vi "Allosense - File to AWS Athena Converter.vi"() -> ()   [LabVIEW 2020]
uses:
  subvis/TimestampAction.ctl
  <vilib>/Utility/file.llb/Read Delimited Spreadsheet (string).vi
  <vilib>/Utility/file.llb/Write Delimited Spreadsheet (string).vi
panel:
  out "Status":string
  in  "Quick Save":bool
  in  "Save Header Settings":bool=TRUE
  in  "Load Header Settings":bool
  in  "Next 2":bool
  in  "Timing":T2(array[cluster])
  in  "Next":bool
  in  "Header Elements":T3(array[cluster])
  in  "Remove Header":bool=TRUE
  in  "Delimiter":string=","
  out "File Contents":string[][](array[string])
  # "Outputs:\n1. Updated .CSV (Timestamp Formatted)\n2. Header Datatype Table .TXT (for AWS Athena)\n3. Saved Header Configurations .BIN"
  # "OPTIONS"
  # "->"
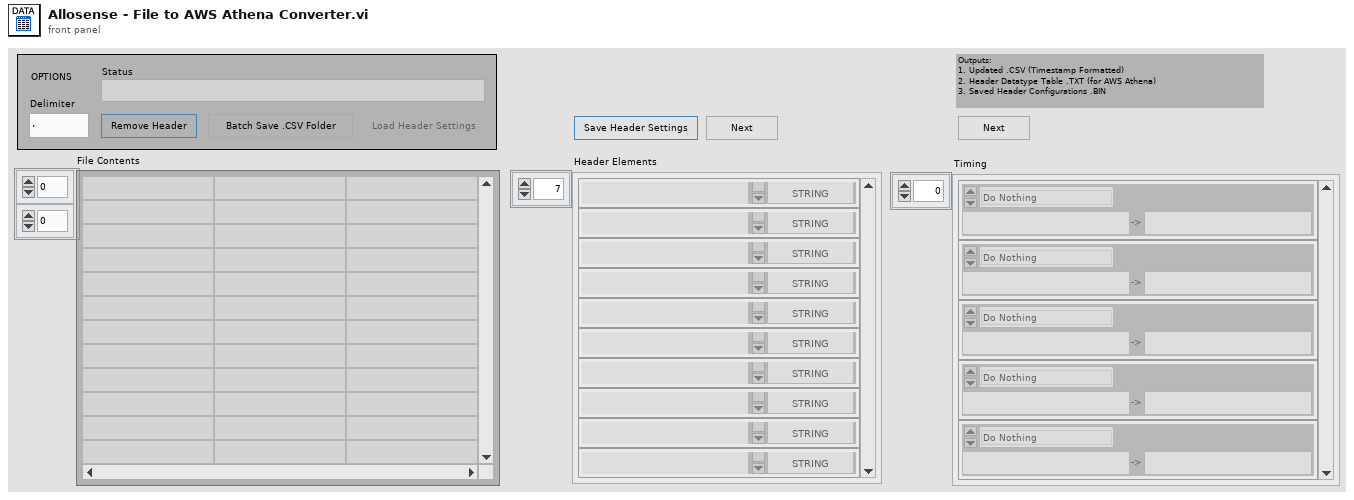
[diagram p1: front panel]
types:
  T1 = typedef "TimestampAction.ctl" = enum16{"Do Nothing", "Remove T"}
  T2 = cluster{"Original":string, "Action":T1, "Processed":string}[]
  T3 = cluster{"Item Name":string, "Item Type":enum16{"STRING", "TINYINT", "SMALLINT", "INT", "BIGINT", "BOOLEAN", "FLOAT", "DOUBLE", "DECIMAL", "ARRAY", "MAP", "TIMESTAMP", "DATE"}}[]
  T4 = enum16{"STRING", "TINYINT", "SMALLINT", "INT", "BIGINT", "BOOLEAN", "FLOAT", "DOUBLE", "DECIMAL", "ARRAY", "MAP", "TIMESTAMP", "DATE"}
  T5 = cluster{"Item Name":string, "Item Type":enum16{"STRING", "TINYINT", "SMALLINT", "INT", "BIGINT", "BOOLEAN", "FLOAT", "DOUBLE", "DECIMAL", "ARRAY", "MAP", "TIMESTAMP", "DATE"}}
  T6 = cluster{"Original":string, "Action":T1, "Processed":string}
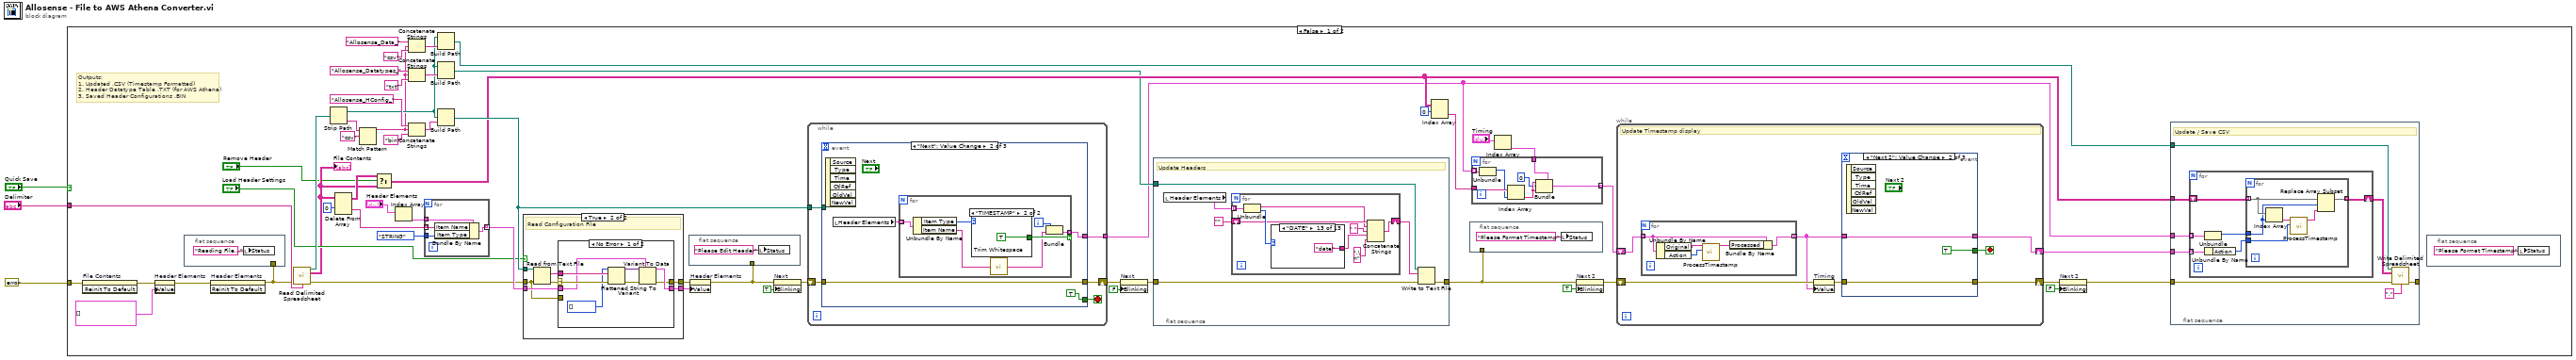
[diagram p0: block diagram]
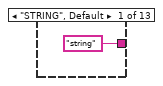
[diagram p2: hidden frame]
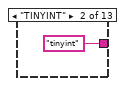
[diagram p3: hidden frame]
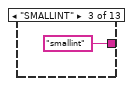
[diagram p4: hidden frame]
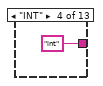
[diagram p5: hidden frame]
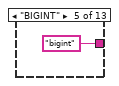
[diagram p6: hidden frame]
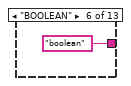
[diagram p7: hidden frame]
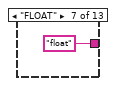
[diagram p8: hidden frame]
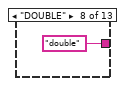
[diagram p9: hidden frame]
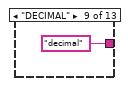
[diagram p10: hidden frame]
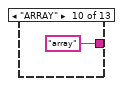
[diagram p11: hidden frame]
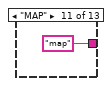
[diagram p12: hidden frame]
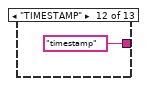
[diagram p13: hidden frame]
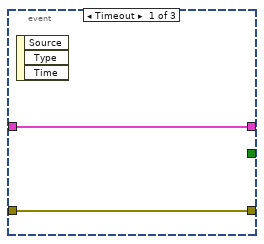
[diagram p14: hidden frame]
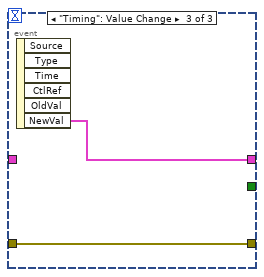
[diagram p15: hidden frame]
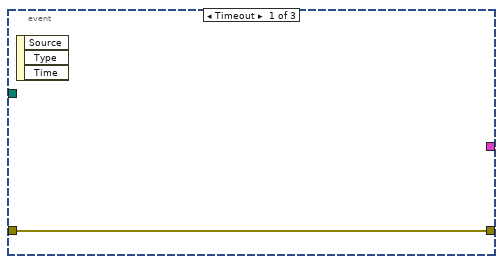
[diagram p16: hidden frame]
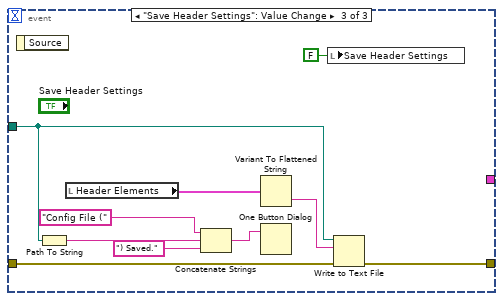
[diagram p18: hidden frame]
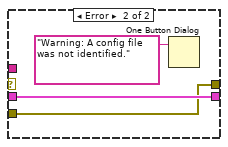
[diagram p20: hidden frame]
diagram:
  n1 = case shown="False" "Quick Save" {
    tunnel: errorcluster {"status"=FALSE, "code"=0, "source"=""} ("error in (no error)") -> [w8 w197]
    tunnel: "Delimiter" -> [w7 w189]
    frame False {
      # "Outputs:\n1. Updated .CSV (Timestamp Formatted)\n2. Header Datatype Table .TXT (for AWS Athena)\n3. Saved Header Configurations .BIN"
      n2 = invoke on="File Contents" class="Arr (strict)" method="Reinit To Default"(error in=w8) -> (error out=w57:errorcluster)  [unwired: 2 in, 2 out]
      n3 = property on="Header Elements" class="Arr (strict)"(error in=w57, "Value"=T3 [] ("Header Elements")) -> (error out=w56:errorcluster)  [unwired: 1 in, 1 out]
      n4 = flat-sequence {
        tunnel: w6 -> [_]
        frame #0 {
          n5 = local write "Status"("Reading File..." ("Status")) -> ()
        }
      }
      n6 = invoke on="Header Elements" class="Arr (strict)" method="Reinit To Default"(error in=w56) -> (error out=w6:errorcluster)  [unwired: 2 in, 2 out]
      n7 = call-poly <vilib>:"Read Delimited Spreadsheet.vi"("error in (no error)"=w6, "delimiter (\\t)"=w7) -> ("new file path (Not A Path if cancelled)"=w49:path, "all rows"=w31:string[][], "error out"=w45:errorcluster)  [unwired: 8 in, 3 out]
      "File Contents" <- w31
      n8 = Strip Path(path=w49) -> (stripped path=w35:path, name=w48:string)
      n9 = Delete From Array(array=w31, index (row)=0) -> (deleted portion=w58:string[], array with subset deleted=w32:string[][])  [unwired: 2 in]
      n10 = Match Pattern(string=w48, regular expression="csv") -> (before substring=w34:string)  [unwired: 1 in, 3 out]
      n11 = Select(t=w32, s="Remove Header", f=w31) -> (s? t:f=w29:string[][])
      n12 = Index Array(array="Header Elements") -> (element=w53:T5)  [unwired: 1 in]
      n13 = Concatenate Strings("Allosense_Data_" ("string"), w34, "csv" ("string")) -> (w38:string)
      n14 = Concatenate Strings("Allosense_Datatypes_" ("string"), w34, "txt" ("string")) -> (w39:string)
      n15 = Concatenate Strings("Allosense_HConfig_" ("string"), w34, "bin" ("string")) -> (w50:string)
      n16 = for {
        tunnel: w58 -> [w187] mode=indexing
        tunnel: w53 -> [w188]
        tunnel: [w186] -> w52 mode=indexing
        tunnel: T4."STRING" ("Item Type") -> [w185]
        n17 = Bundle By Name(cluster=w188, "Item Name"=w187, "Item Type"=w185) -> (w186:T5)
      }
      n18 = Build Path(base path=w35, name or relative path=w38) -> (appended path=w33:path)
      n19 = Build Path(base path=w35, name or relative path=w39) -> (appended path=w28:path)
      n20 = Build Path(base path=w35, name or relative path=w50) -> (appended path=w46:path)
      n21 = case shown="True" "Load Header Settings" {
        tunnel: w52 -> [w166 w170]
        tunnel: [w166 w169] -> w22
        tunnel: w46 -> [_ w173]
        tunnel: w45 -> [w165 w167]
        tunnel: [w165 w168] -> w21
        frame False {
          # "Continue"
        }
        frame True {
          # "Read Configuration File"
          n22 = Read from Text File(file (use dialog)=w173, error in=w167) -> (text=w171:string, error out=w172:errorcluster)  [unwired: 2 in, 2 out]
          n23 = case shown="No Error" w172 {
            selector: w172 -> [w180 _]
            tunnel: w171 -> [w181 _]
            tunnel: w170 -> [w178 w184]
            tunnel: [w176 w184] -> w169
            tunnel: [w175 w182] -> w168
            tunnel: w167 -> [_ w182]
            frame No Error {
              n24 = Flattened String To Variant(4:w180, 6:w181, 7:i16[] [] ("type string")) -> (0:w179:errorcluster, 3:w177:variant)
              n25 = Variant To Data(error in=w179, type=w178, Variant=w177) -> (data=w176:T3, error out=w175:errorcluster)
            }
            frame Error {
              n26 = One Button Dialog(message="Warning: A config file was not identified.") -> ()  [unwired: 1 in, 1 out]
            }
          }
        }
      }
      n27 = flat-sequence {
        tunnel: w5 -> [_]
        frame #0 {
          n28 = local write "Status"("Please Edit Header" ("Status")) -> ()
        }
      }
      n29 = property on="Header Elements" class="Arr (strict)"(error in=w21, "Value"=w22) -> (error out=w5:errorcluster)  [unwired: 1 in, 1 out]
      n30 = property on="Next" class="Bool"(error in=w5, "Blinking"=TRUE) -> (error out=w18:errorcluster)  [unwired: 1 in, 1 out]
      n31 = while {
        tunnel: [w134] -> w19
        tunnel: w46 -> [w131]
        shift-right: [w132] -> w14
        shift-left: w18 -> [w133]
        stop <- w130 stop-if-true
        n32 = event shown="[1] \"Next\": Value Change" {
          selector: _ -> [_ _ _]
          dyn-events: _ -> [_ _ _]
          timeout: _ -> [_ _ _]
          tunnel: [_ w139 _] -> w134
          tunnel: w133 -> [w135 w137 w156]
          tunnel: [w135 w137 w155] -> w132
          tunnel: w131 -> [_ _ w154]
          tunnel: [_ TRUE _] -> w130
          event Timeout {
            n33 = event-data() -> ()  [unwired: 1 in, 3 out]
          }
          event "Next": Value Change {
            n34 = event-data() -> ()  [unwired: 1 in, 6 out]
            n35 = local read "Header Elements"() -> (w138:T3)
            n36 = for {
              tunnel: w138 -> [w146] mode=indexing
              tunnel: [w143] -> w139 mode=indexing if=w144
              i -> [w142]
              n37 = Unbundle By Name(w146) -> ("Item Type"=w145:T4, "Item Name"=w141:string)
              n38 = case shown="\"TIMESTAMP\"" w145 {
                tunnel: [_ TRUE] -> w144
                frame Default {
                }
                frame "TIMESTAMP" {
                }
              }
              n39 = call <vilib>:"Trim Whitespace.vi"("string"=w141) -> ("trimmed string"=w140:string)  [unwired: 1 in]
              n40 = Bundle(w142, "trimmed string"=w140) -> (w143:cluster{i32, "trimmed string":string})  [unwired: 1 in]
            }
          }
          event "Save Header Settings": Value Change {
            n41 = event-data() -> ()  [unwired: 1 in, 1 out]
            n42 = Path To String(path=w154) -> (string=w153:string)
            n43 = local read "Header Elements"() -> (w148:T3)
            n44 = Concatenate Strings("Config File (" ("message"), w153, ") Saved." ("string")) -> (w150:string)
            n45 = Variant To Flattened String(Variant=w148) -> (data string=w157:string)  [unwired: 1 out]
            n46 = One Button Dialog(message=w150) -> ()  [unwired: 1 in, 1 out]
            n47 = local write "Save Header Settings"(FALSE ("Save Header Settings")) -> ()
            n48 = Write to Text File(file (use dialog)=w154, text=w157, error in=w156) -> (error out=w155:errorcluster)  [unwired: 1 in, 2 out]
          }
        }
      }
      n49 = property on="Next" class="Bool"(error in=w14, "Blinking"=FALSE) -> (error out=w15:errorcluster)  [unwired: 1 in, 1 out]
      n50 = flat-sequence {
        tunnel: w15 -> [w66]
        tunnel: [w65] -> w4
        tunnel: w28 -> [w67]
        frame #0 {
          # "Update Headers"
          n51 = local read "Header Elements"() -> (w69:T3)
          n52 = for {
            tunnel: w69 -> [w77] mode=indexing
            shift-right: [w75] -> w64
            shift-left: "" ("Item Name") -> [w74]
            n53 = Unbundle(w77) -> ("Item Name"=w73:string, "Item Type"=w76:T4)
            n54 = case shown="\"DATE\"" w76 {
              tunnel: ["string" ("Item Name") "tinyint" ("Item Name") "smallint" ("Item Name") "int" ("Item Name") "bigint" ("Item Name") "boolean" ("Item Name") "float" ("Item Name") "double" ("Item Name") "decimal" ("Item Name") "array" ("Item Name") "map" ("Item Name") "timestamp" ("Item Name") "date" ("Item Name")] -> w71
              frame "STRING", Default {
              }
              frame "TINYINT" {
              }
              frame "SMALLINT" {
              }
              frame "INT" {
              }
              frame "BIGINT" {
              }
              frame "BOOLEAN" {
              }
              frame "FLOAT" {
              }
              frame "DOUBLE" {
              }
              frame "DECIMAL" {
              }
              frame "ARRAY" {
              }
              frame "MAP" {
              }
              frame "TIMESTAMP" {
              }
              frame "DATE" {
              }
            }
            n55 = Concatenate Strings(w74, w73, " " ("string"), w71, ",\n" ("string")) -> (w75:string)
          }
          n56 = Write to Text File(file (use dialog)=w67, text=w64, error in=w66) -> (error out=w65:errorcluster)  [unwired: 1 in, 2 out]
        }
      }
      n57 = Index Array(array=w29, index (row)=0) -> (element=w23:string[])  [unwired: 1 in]
      n58 = flat-sequence {
        tunnel: w4 -> [_]
        frame #0 {
          n59 = local write "Status"("Please Format Timestamp" ("Status")) -> ()
        }
      }
      n60 = Index Array(array="Timing") -> (element=w26:T6)  [unwired: 1 in]
      n61 = for {
        tunnel: w26 -> [w164]
        tunnel: w19 -> [w163] mode=indexing
        tunnel: [w162] -> w25 mode=indexing
        tunnel: w23 -> [w161]
        n62 = Unbundle(w163) -> (w160:i32)  [unwired: 1 out]
        n63 = Index Array(array=w161, index=w160) -> (element=w159:string)
        n64 = Bundle(cluster=w164, "Original"=w159, "Action"=0, "Processed"=w159) -> (w162:T6)
      }
      n65 = property on="Next 2" class="Bool"(error in=w4, "Blinking"=TRUE) -> (error out=w13:errorcluster)  [unwired: 1 in, 1 out]
      n66 = while {
        shift-right: [w116] -> w20
        shift-left: w25 -> [w114]
        shift-right: [w111] -> w10
        shift-left: w13 -> [w115]
        stop <- w117 stop-if-true
        # "Update Timestamp display"
        n67 = for {
          tunnel: w114 -> [w122] mode=indexing
          tunnel: [w121] -> w113 mode=indexing
          n68 = Unbundle By Name(w122) -> ("Original"=w120:string, "Action"=w119:T1)
          n69 = call "ProcessTimestamp.vi"("Action"=w119, "Original"=w120) -> ("Processed"=w118:string)  [unwired: 9 in]
          n70 = Bundle By Name(cluster=w122, "Processed"=w118) -> (w121:T6)
        }
        n71 = property on="Timing" class="Arr (strict)"(error in=w115, "Value"=w113) -> (error out=w112:errorcluster)  [unwired: 1 in, 1 out]
        n72 = event shown="[1] \"Next 2\": Value Change" {
          selector: _ -> [_ _ _]
          dyn-events: _ -> [_ _ _]
          timeout: _ -> [_ _ _]
          tunnel: [_ TRUE _] -> w117
          tunnel: [w124 w126 w129] -> w116
          tunnel: w113 -> [w124 w126 _]
          tunnel: w112 -> [w123 w125 w128]
          tunnel: [w123 w125 w128] -> w111
          event Timeout {
            n73 = event-data() -> ()  [unwired: 1 in, 3 out]
          }
          event "Next 2": Value Change {
            n74 = event-data() -> ()  [unwired: 1 in, 6 out]
          }
          event "Timing": Value Change {
            n75 = event-data() -> ("NewVal"=w129:T2)  [unwired: 1 in, 5 out]
          }
        }
      }
      n76 = property on="Next 2" class="Bool"(error in=w10, "Blinking"=FALSE) -> (error out=w9:errorcluster)  [unwired: 1 in, 1 out]
      n77 = flat-sequence {
        tunnel: w9 -> [w93]
        tunnel: w20 -> [w98]
        tunnel: w33 -> [w95]
        tunnel: w29 -> [w96]
        tunnel: w19 -> [w97]
        tunnel: [w91] -> _
        frame #0 {
          # "Update / Save CSV"
          n78 = for {
            tunnel: w98 -> [w104] mode=indexing
            tunnel: w97 -> [w103] mode=indexing
            shift-right: [w99] -> w94
            shift-left: w96 -> [w102]
            n79 = Unbundle By Name(w104) -> ("Action"=w100:T1)
            n80 = Unbundle(w103) -> (w101:i32)  [unwired: 1 out]
            n81 = for {
              tunnel: w102 -> [w110] mode=indexing
              tunnel: w101 -> [w109]
              tunnel: w100 -> [w106]
              tunnel: [w105] -> w99 mode=indexing
              n82 = Index Array(array=w110, index=w109) -> (element=w108:string)
              n83 = call "ProcessTimestamp.vi"("Action"=w106, "Original"=w108) -> ("Processed"=w107:string)  [unwired: 9 in]
              n84 = Replace Array Subset(array=w110, new element=w107, index=w109) -> (w105:string[])
            }
          }
          n85 = call-poly <vilib>:"Write Delimited Spreadsheet.vi"("file path (dialog if empty)"=w95, "2D data"=w94, "error in (no error)"=w93, "delimiter (\\t)"="," ("delimiter (\\t)")) -> ("error out"=w91:errorcluster)  [unwired: 10 in, 1 out]
        }
      }
      n86 = flat-sequence {
        frame #0 {
          n87 = local write "Status"("Please Format Timestamp" ("Status")) -> ()
        }
      }
    }
    frame True {
      n88 = call "File Dialog"("prompt"="Select a folder containing .csv's.", "error in"=w197) -> ("selected path"=w195:path, "error out"=w194:errorcluster)  [unwired: 10 in, 2 out]
      n89 = call <vilib>:"Recursive File List.vi"("error in (no error)"=w194, "Folder Path"=w195) -> ("error out"=w192:errorcluster, "All Files in Dir"=w193:path[])  [unwired: 5 in, 3 out]
      n90 = for {
        tunnel: w193 -> [w219] mode=indexing
        shift-right: [w220] -> w190
        shift-left: w192 -> [w221]
        tunnel: [w219] -> w191 mode=indexing if=w218
        # "Select only CSV Files"
        n91 = Strip Path(path=w219) -> (name=w224:string)  [unwired: 1 out]
        n92 = Search and Replace String(input string=w224, search string=".csv", error in=w221) -> (offset past replacement=w222:i32, error out=w220:errorcluster)  [unwired: 5 in, 2 out]
        n93 = Greater Or Equal To 0?(x=w222) -> (x >= 0?=w218:bool)
      }
      n94 = for {
        N -> [w203]
        tunnel: w191 -> [w208] mode=indexing
        tunnel: w190 -> [w214]
        tunnel: w189 -> [w213]
        i -> [w207]
        n95 = call-poly <vilib>:"Read Delimited Spreadsheet.vi"("file path (dialog if empty)"=w208, "error in (no error)"=w214, "delimiter (\\t)"=w213) -> ("all rows"=w210:string[][], "error out"=w211:errorcluster)  [unwired: 7 in, 4 out]
        n96 = in-place {
          n97 = in-place-match #1(w210) -> (w216:string[][])
          n98 = Delete From Array(array=w216, index (row)=0) -> (array with subset deleted=w215:string[][])  [unwired: 2 in, 1 out]
          n99 = in-place-match #1(w215) -> (w209:string[][])
        }
        n100 = Number To Decimal String(number=w203) -> (decimal integer string=w202:string)  [unwired: 1 in]
        n101 = Number To Decimal String(number=w207) -> (decimal integer string=w205:string)  [unwired: 1 in]
        n102 = Concatenate Strings("Processing " ("name"), w205, " out of " ("string"), w202, " files. Filename: " ("string")) -> (w200:string)
        n103 = call-poly <vilib>:"Write Delimited Spreadsheet.vi"("file path (dialog if empty)"=w208, "2D data"=w209, "error in (no error)"=w211, "delimiter (\\t)"="," ("delimiter (\\t)")) -> ()  [unwired: 10 in, 2 out]
        n104 = Strip Path(path=w208) -> (name=w199:string)  [unwired: 1 out]
        n105 = Concatenate Strings(w200, w199) -> (→"Status":string)
      }
    }
  }
